vi "log message.vi"(8 "error in (no error)":errorcluster, 9 "message type":string(combo)="[INFO]", 10 "Message to log":string, 11 "Log File in":refnum<class "CM_Log File.lvclass">) -> (0 "error out":errorcluster, 3 "Log File out":refnum<class "CM_Log File.lvclass">)   [LabVIEW 2018, in "CM_Log File.lvclass"]
uses:
  CM_Log File.lvclass
  CM_Log File.lvclass/CM_Log File.ctl
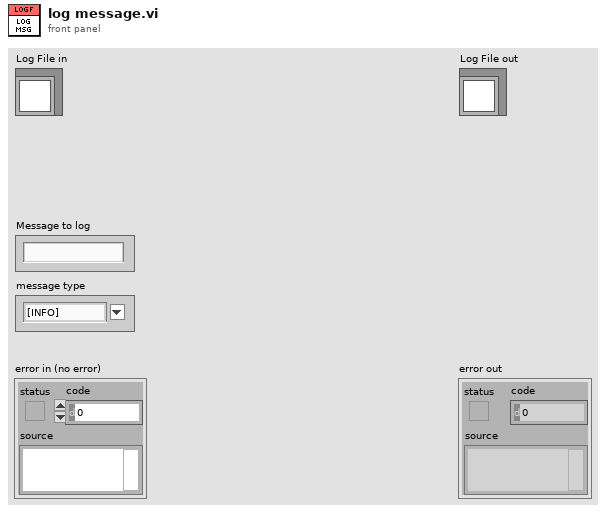
[diagram p1: front panel]
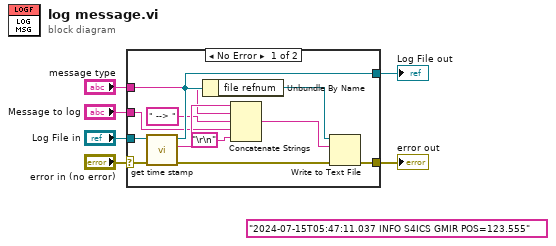
[diagram p0: block diagram]
diagram:
  (unwired) "2024-07-15T05:47:11.037 INFO S4ICS GMIR POS=123.555" ("string")
  n1 = case shown="No Error" "error in (no error)" {
    selector: "error in (no error)" -> [w10 w20]
    tunnel: [w18 w20] -> w5
    tunnel: [w14 w19] -> w3
    tunnel: "Log File in" -> [w9 w19]
    tunnel: "Message to log" -> [w8 _]
    tunnel: "message type" -> [w7 _]
    frame No Error {
      n2 = call "get time stamp.vi"("error in (no error)"=w10, "Log File in"=w9) -> ("error out"=w13:errorcluster, "time stamp"=w12:string, "Log File out"=w14:refnum<class "CM_Log File.lvclass">)  [unwired: 7 in]
      n3 = Unbundle By Name(w14) -> ("file refnum"=w17:refnum<file>)
      n4 = Concatenate Strings(w12, w7, " --> " ("string"), w8, "\r\n") -> (w15:string)
      n5 = Write to Text File(file (use dialog)=w17, text=w15, error in=w13) -> (error out=w18:errorcluster)  [unwired: 1 in, 2 out]
    }
    frame Error {
    }
  }
  "error out" <- w5
  "Log File out" <- w3
